vi "MatrixAlgorithm.vi"() -> ()   [LabVIEW 2011]
panel:
  out "ApplyElement":dbl
  out "Current col":i32
  out "Sweep":i32
  out "row state":i32[](array[numeric])
  out "Num elements in col":i32[](array[numeric])
  in  "Array In":dbl[][](array[numeric])
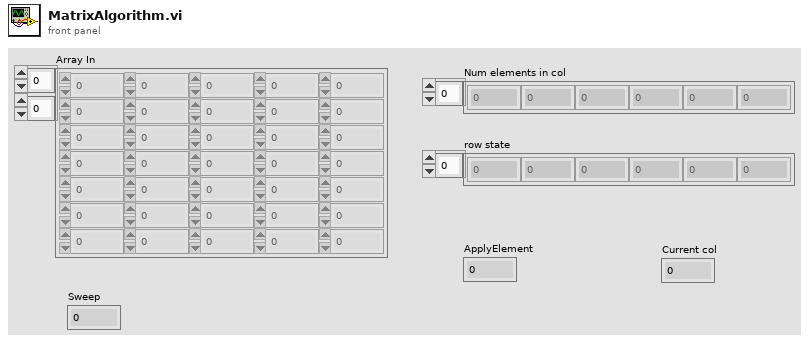
[diagram p1: front panel]
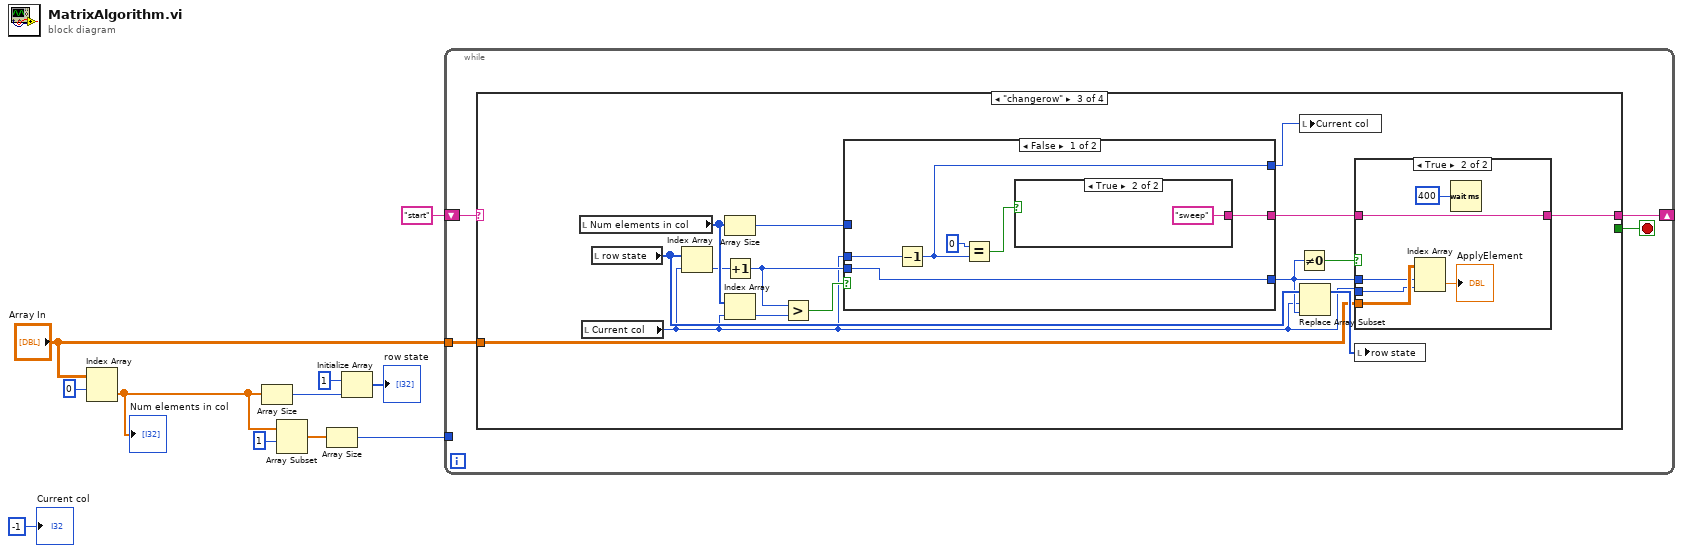
[diagram p0: block diagram]
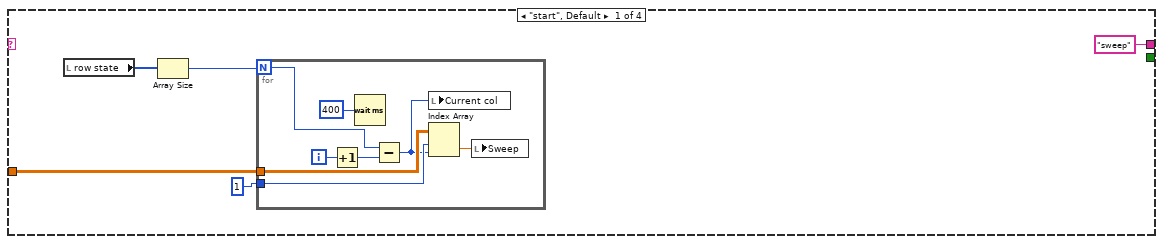
[diagram p2: hidden frame]
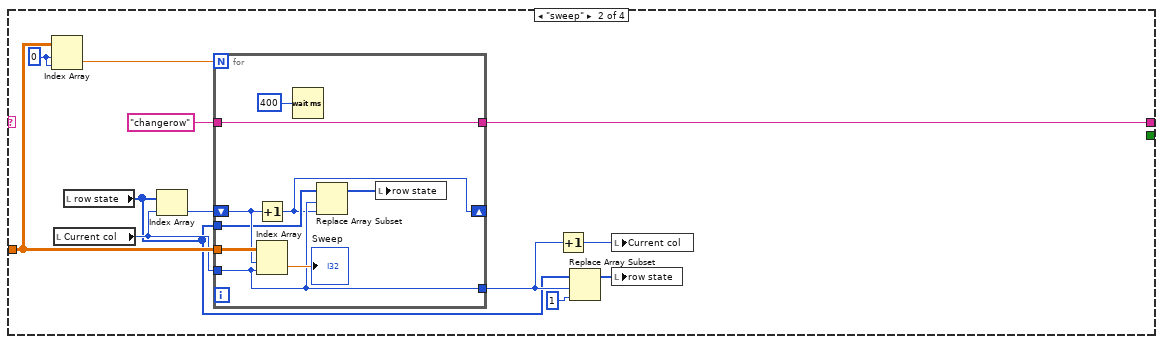
[diagram p3: hidden frame]
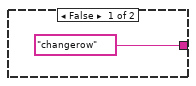
[diagram p5: hidden frame]
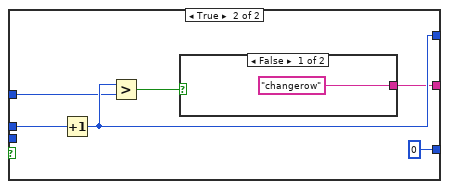
[diagram p6: hidden frame]
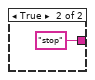
[diagram p7: hidden frame]
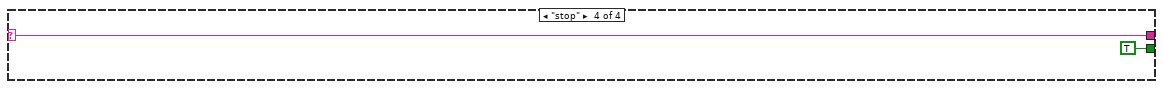
[diagram p8: hidden frame]
diagram:
  n1 = Index Array(array="Array In", index (row)=0) -> (element=w6:dbl[])  [unwired: 1 in]
  "Num elements in col" <- w6
  n2 = Array Size(array=w6) -> (size(s)=w7:i32)
  n3 = Array Subset(array=w6, index=1) -> (w9:dbl[])  [unwired: 1 in]
  n4 = Array Size(array=w9) -> (size(s)=w4:i32)
  n5 = Initialize Array(1, w7) -> (→"row state":i32[])
  n6 = while {
    tunnel: w4 -> [_]
    shift-right: [w14] -> _
    shift-left: "start" -> [w15]
    tunnel: "Array In" -> [w13]
    stop <- w12 stop-if-true
    n7 = case shown="\"changerow\"" w15 {
      selector: w15 -> [_ _ _ w89]
      tunnel: ["sweep" w33 w55 w89] -> w14
      tunnel: w13 -> [w16 w36 w53 _]
      tunnel: [_ _ _ TRUE] -> w12
      frame "start", Default {
        n8 = local read "row state"() -> (w19:i32[])
        n9 = Array Size(array=w19) -> (size(s)=w18:i32)
        n10 = for {
          N: w18 -> [w26]
          tunnel: 1 -> [w27]
          tunnel: w16 -> [w28]
          i -> [w25]
          n11 = Increment(x=w25) -> (x+1=w24:i32)
          n12 = Wait (ms)(milliseconds to wait=u32 400) -> ()  [unwired: 1 out]
          n13 = Subtract(x=w26, y=w24) -> (x-y=w22:i32)
          n14 = local write "Current col"(w22) -> ()
          n15 = Index Array(array=w28, index (row)=w27, index (col)=w22) -> (element=w21:dbl)
          n16 = local write "Sweep"(w21) -> ()
        }
      }
      frame "sweep" {
        w40 = 0 ("index")
        n17 = Index Array(array=w36, index (row)=w40, index (col)=w40) -> (element=w39:dbl)
        n18 = local read "Current col"() -> (w35:i32)
        n19 = local read "row state"() -> (w29:i32[])
        n20 = Index Array(array=w29, index=w35) -> (element=w37:i32)
        n21 = for {
          N: w39 -> [_]
          tunnel: [w48] -> w33
          tunnel: "changerow" -> [w48]
          tunnel: w35 -> [w43]
          tunnel: w36 -> [w47]
          tunnel: [w43] -> w31
          shift-right: [w42] -> _
          shift-left: w37 -> [w45]
          tunnel: w29 -> [w44]
          n22 = Increment(x=w45) -> (x+1=w42:i32)
          n23 = Index Array(array=w47, index (row)=w45, index (col)=w43) -> (element=→"Sweep":dbl)
          n24 = Wait (ms)(milliseconds to wait=u32 400) -> ()  [unwired: 1 out]
          n25 = Replace Array Subset(array=w44, new element=w42, index=w43) -> (w41:i32[])
          n26 = local write "row state"(w41) -> ()
        }
        n27 = Increment(x=w31) -> (x+1=w34:i32)
        n28 = Replace Array Subset(array=w29, new element=1 ("new element/subarray"), index=w31) -> (w32:i32[])
        n29 = local write "Current col"(w34) -> ()
        n30 = local write "row state"(w32) -> ()
      }
      frame "changerow" {
        n31 = local read "Num elements in col"() -> (w60:i32[])
        n32 = local read "Current col"() -> (w50:i32)
        n33 = local read "row state"() -> (w62:i32[])
        n34 = Index Array(array=w62, index=w50) -> (element=w58:i32)
        n35 = Array Size(array=w60) -> (size(s)=w59:i32)
        n36 = Increment(x=w58) -> (x+1=w57:i32)
        n37 = Index Array(array=w60, index=w50) -> (element=w64:i32)
        n38 = Greater?(x=w57, y=w64) -> (0:w63:bool)
        n39 = case shown="False" w63 {
          tunnel: [w77 0] -> w51
          tunnel: w57 -> [w77 _]
          tunnel: [w75 w83] -> w52
          tunnel: [w72 w80] -> w56
          tunnel: w50 -> [w76 w84]
          tunnel: w59 -> [_ w82]
          frame False {
            n40 = Decrement(x=w76) -> (x-1=w75:i32)
            n41 = Equal?(x=0, y=w75) -> (x = y?=w73:bool)
            n42 = case shown="True" w73 {
              tunnel: ["changerow" "sweep"] -> w72
              frame False {
              }
              frame True {
              }
            }
          }
          frame True {
            n43 = Increment(x=w84) -> (x+1=w83:i32)
            n44 = Greater?(x=w83, y=w82) -> (0:w81:bool)
            n45 = case shown="False" w81 {
              tunnel: ["changerow" "stop"] -> w80
              frame False {
              }
              frame True {
              }
            }
          }
        }
        n46 = Not Equal To 0?(x=w51) -> (x != 0?=w54:bool)
        n47 = local write "Current col"(w52) -> ()
        n48 = Replace Array Subset(array=w62, new element=w51, index=w50) -> (w61:i32[])
        n49 = case shown="True" w54 {
          tunnel: w56 -> [w65 w71]
          tunnel: [w65 w71] -> w55
          tunnel: w53 -> [_ w70]
          tunnel: w50 -> [_ w69]
          tunnel: w51 -> [_ w68]
          frame False {
          }
          frame True {
            n50 = Index Array(array=w70, index (row)=w68, index (col)=w69) -> (element=→"ApplyElement":dbl)
            n51 = Wait (ms)(milliseconds to wait=u32 400) -> ()  [unwired: 1 out]
          }
        }
        n52 = local write "row state"(w61) -> ()
      }
      frame "stop" {
      }
    }
  }
  "Current col" <- -1 ("Current col")
